vi "Extract Analog TTL Transitions Sample.vi"() -> ()   [LabVIEW 2009]
uses:
  <vilib>/Waveform/DTblOps.llb/DTbl Analog to Digital.vi
  <vilib>/Utility/file.llb/Write To Spreadsheet File (DBL).vi
panel:
  in  "Path":path=path "F:/data/tomo/simttl-5Mhz.txt"
  in  "Frequency":dbl=40.0
  out "subarray":u32[](array[numeric])
  in  "Phase":dbl(knob) scale=-180.0..180.0
  out "Falling Transition":u32[](array[numeric])
  out "Rising Transition":u32[](array[numeric])
  out "odd array":u32[][](array[numeric])
  out "even array":u32[][](array[numeric])
  out "digital data 2":digitaldata
  out "Array 3":dbl[](array[numeric])
  out "Array":dbl[](array[numeric])
  out "Square with Uniform Noise":dynamicdata(graph)
  in  "stop":bool
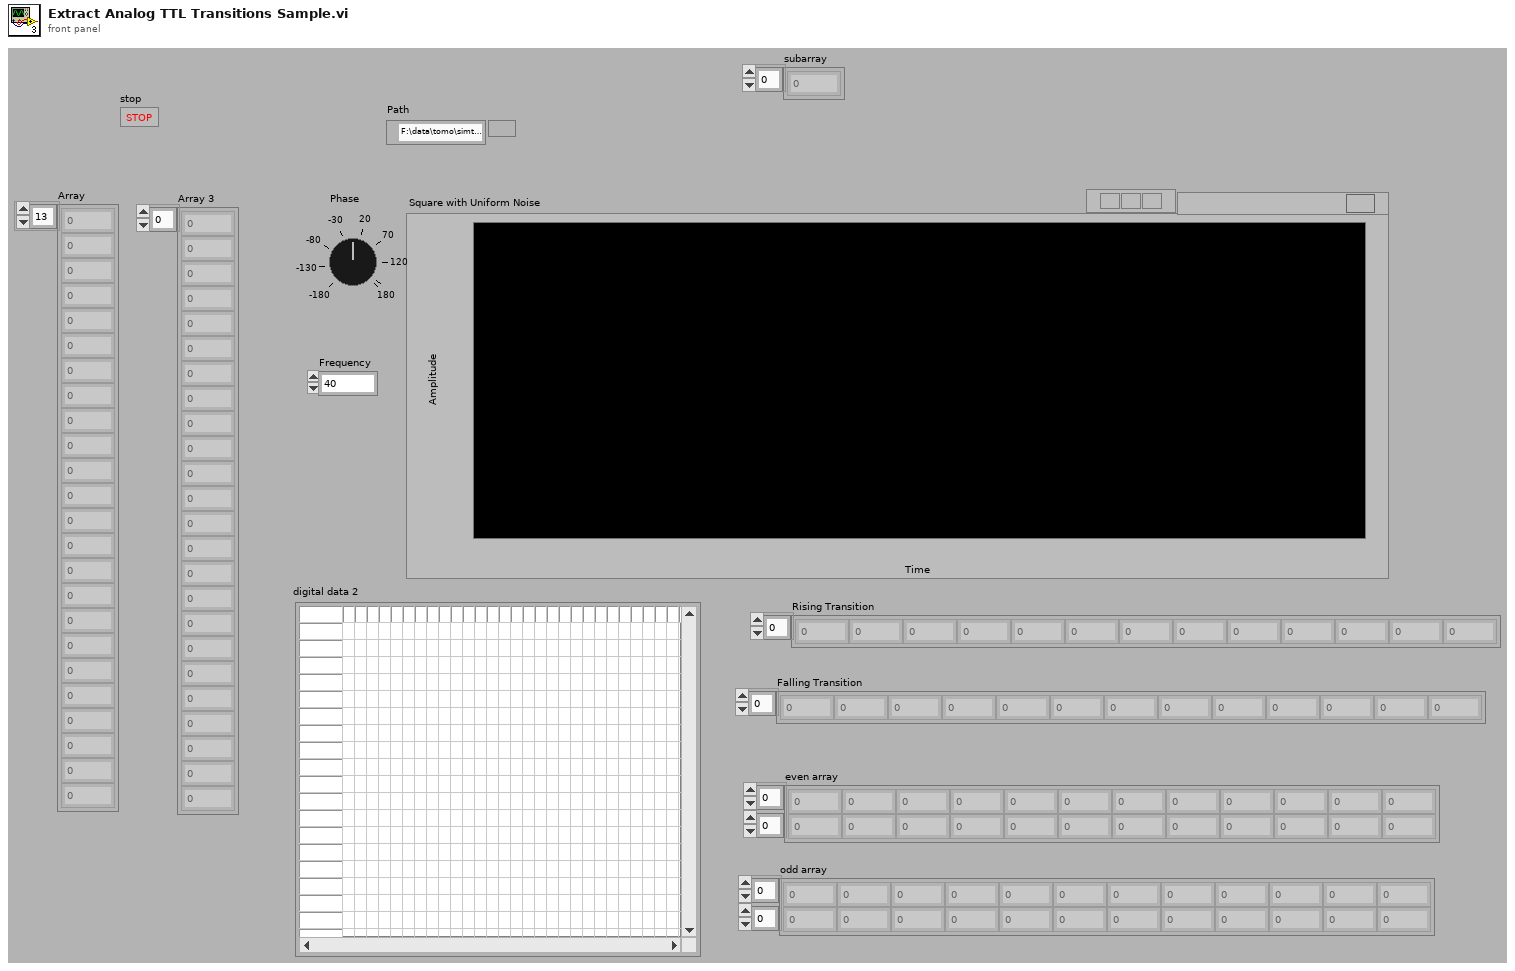
[diagram p1: front panel]
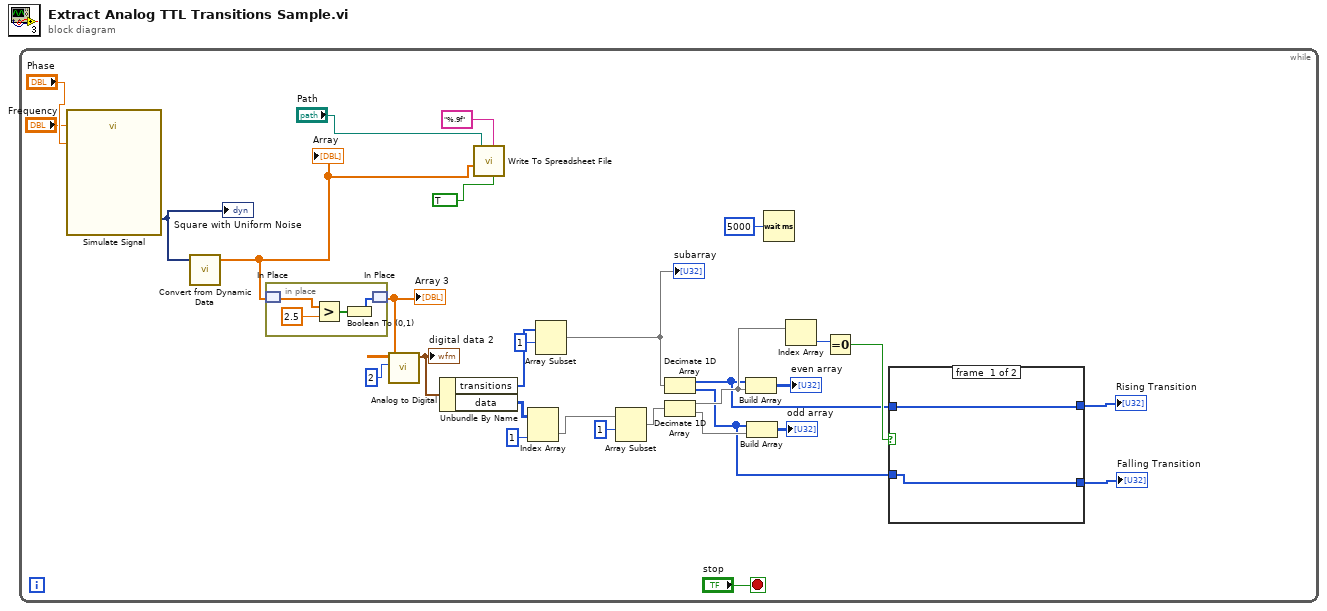
[diagram p0: block diagram]
diagram:
  n1 = while {
    stop <- "stop" stop-if-true
    n2 = call "Simulate Signal"("Frequency"="Frequency", "Phase"="Phase") -> ("Square with Uniform Noise"=w28:dynamicdata)  [unwired: 12 in, 1 out]
    "Square with Uniform Noise" <- w28
    n3 = call "Convert from Dynamic Data"("Dynamic Data Type"=w28) -> ("Array"=w4:dbl[])  [unwired: 3 in]
    "Array" <- w4
    n4 = in-place {
      n5 = in-place-match #1(w4) -> (w36:dbl[])
      n6 = Greater?(x=w36, y=2.5) -> (0:w38:bool[])
      n7 = Boolean To (0,1)(Boolean=w38) -> (0, 1=w35:i16[])
      n8 = in-place-match #1(w35) -> (w25:dbl[])
    }
    "Array 3" <- w25
    n9 = call-poly <vilib>:"Analog to Digital.vi"("resolution (16 bit)"=2, "analog waveform"=w25) -> ("digital data"=w26:digitaldata)  [unwired: 6 in, 3 out]
    "digital data 2" <- w26
    n10 = Unbundle By Name(w26) -> ("transitions"=w11:u32[], "data"=w24:u8[][])
    n11 = call-poly <vilib>:"Write To Spreadsheet File.vi"("transpose? (no:F)"=TRUE ("append to file? (new file:F)"), "format (%.3f)"="%.9f", "1D data"=w4, "file path (dialog if empty)"="Path") -> ()  [unwired: 4 in, 1 out]
    n12 = Index Array(array=w24, index (col)=1 ("disabled index (col)")) -> (element=w8:u8[])  [unwired: 1 in]
    n13 = Array Subset(array=w11, index=1) -> (w9:u32[])  [unwired: 1 in]
    "subarray" <- w9
    n14 = Array Subset(array=w8, index=1) -> (w7:u8[])  [unwired: 1 in]
    n15 = Decimate 1D Array(w9) -> (w17:u32[], w13:u32[])
    n16 = Decimate 1D Array(w7) -> (w20:u8[], w14:u8[])
    n17 = Build Array(w17, w20) -> (→"even array":u32[][])
    n18 = Build Array(w13, w14) -> (→"odd array":u32[][])
    n19 = Wait (ms)(milliseconds to wait=u32 5000) -> ()  [unwired: 1 out]
    n20 = Index Array(array=w20) -> (element=w19:u8)  [unwired: 1 in]
    n21 = Equal To 0?(x=w19) -> (x = 0?=w18:bool)
    n22 = case shown="True" w18 {
      tunnel: w17 -> [w32 w34]
      tunnel: w13 -> [w31 w33]
      tunnel: [w31 w34] -> w15
      tunnel: [w32 w33] -> w16
      frame #0 {
      }
      frame #1 {
      }
    }
    "Rising Transition" <- w16
    "Falling Transition" <- w15
  }
